vi "Local IP Address.vi"() -> (2 "IP Address":string)   [LabVIEW 2011]
doc: "Gets the IP address of the local machine. If the machine has multiple network adapters, this VI returns the first one.\n\n\nVersion 1.0 - 02/13/2013\n\nPhaeron, Inc.\nwww.phaeron.com\ninfo@phaeron.com"
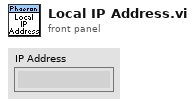
[diagram p1: front panel]
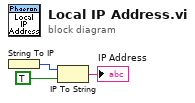
[diagram p0: block diagram]
diagram:
  n1 = String To IP() -> (0:w2:u32)  [unwired: 1 out]
  n2 = IP To String(1:TRUE ("dot notation? (F)"), 2:w2) -> (0:→"IP Address":string)
